vi "位置显示.vi"(5 "right":dbl=1152.0, 7 "left":dbl=846.0, 8 "error in (no error) 2":errorcluster, 10 "簇":T2, 11 "Image in":T1(plugin-control)) -> (0 "error out":errorcluster caption="错误输出", 1 "左":dbl, 2 "右":dbl, 3 "Image out":T1(plugin-control), 4 "x或y？":bool)   [LabVIEW 2017]
panel:
  out "line start X":dbl
  out "x/y":dbl
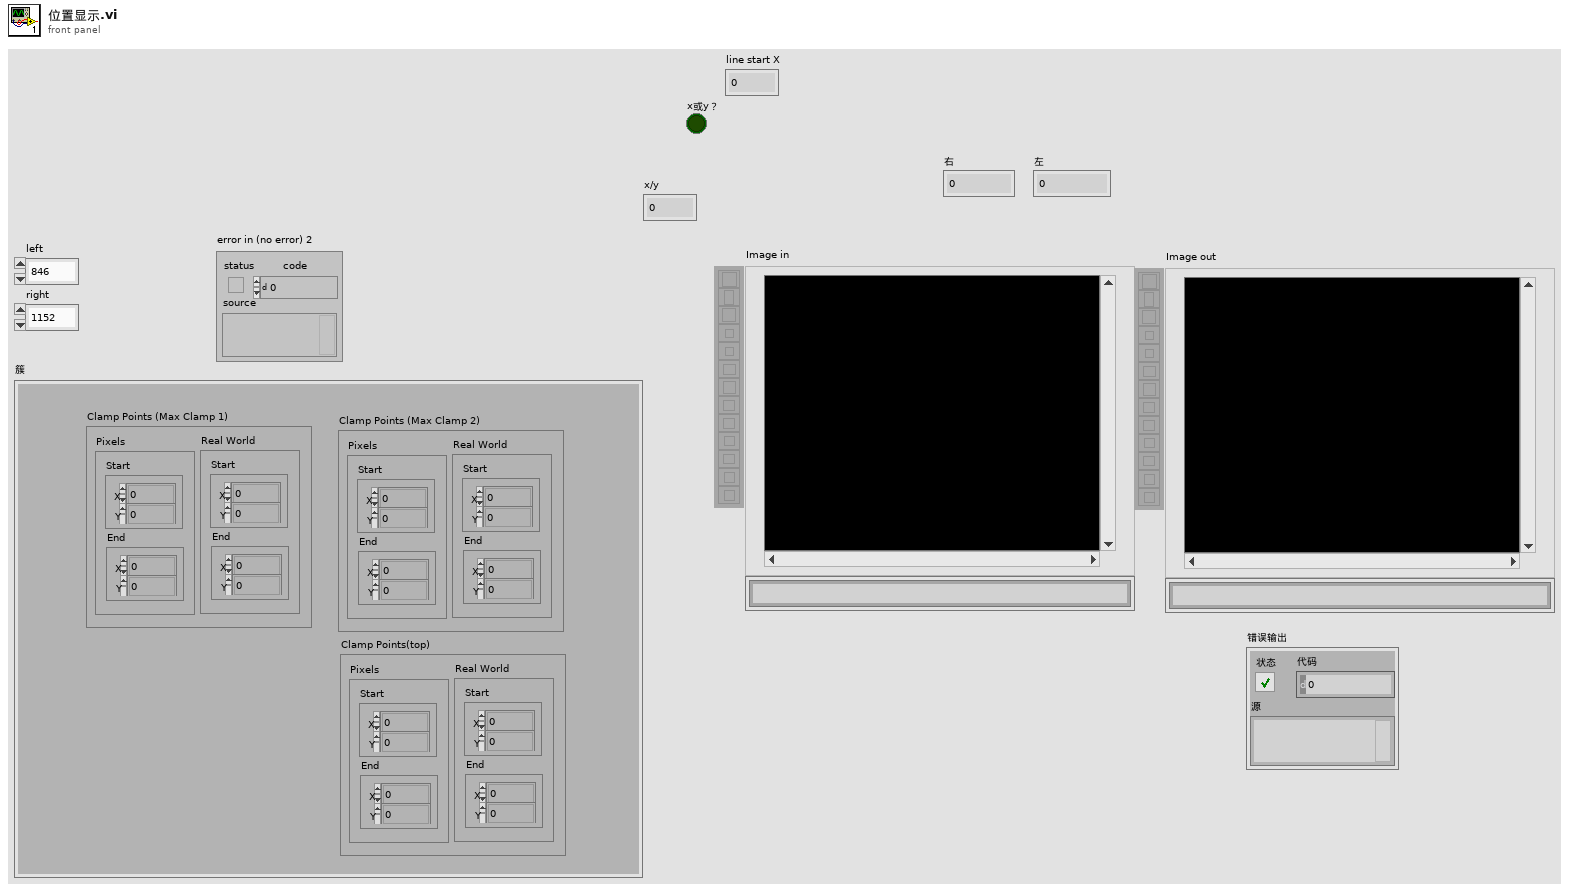
[diagram p1: front panel]
types:
  T1 = typedef "IMAQ Image.ctl" = refnum<image>
  T2 = cluster{"Clamp Points (Max Clamp 1)":cluster{"Pixels ":cluster{"Start":cluster{"X":dbl, "Y":dbl}, "End":cluster{"X":dbl, "Y":dbl}}, "Real World":cluster{"Start":cluster{"X":dbl, "Y":dbl}, "End":cluster{"X":dbl, "Y":dbl}}}, "Clamp Points (Max Clamp 2)":cluster{"Pixels ":cluster{"Start":cluster{"X":dbl, "Y":dbl}, "End":cluster{"X":dbl, "Y":dbl}}, "Real World":cluster{"Start":cluster{"X":dbl, "Y":dbl}, "End":cluster{"X":dbl, "Y":dbl}}}, "Clamp Points(top)":cluster{"Pixels ":cluster{"Start":cluster{"X":dbl, "Y":dbl}, "End":cluster{"X":dbl, "Y":dbl}}, "Real World":cluster{"Start":cluster{"X":dbl, "Y":dbl}, "End":cluster{"X":dbl, "Y":dbl}}}}
  T3 = cluster{"Pixels ":cluster{"Start":cluster{"X":dbl, "Y":dbl}, "End":cluster{"X":dbl, "Y":dbl}}, "Real World":cluster{"Start":cluster{"X":dbl, "Y":dbl}, "End":cluster{"X":dbl, "Y":dbl}}}
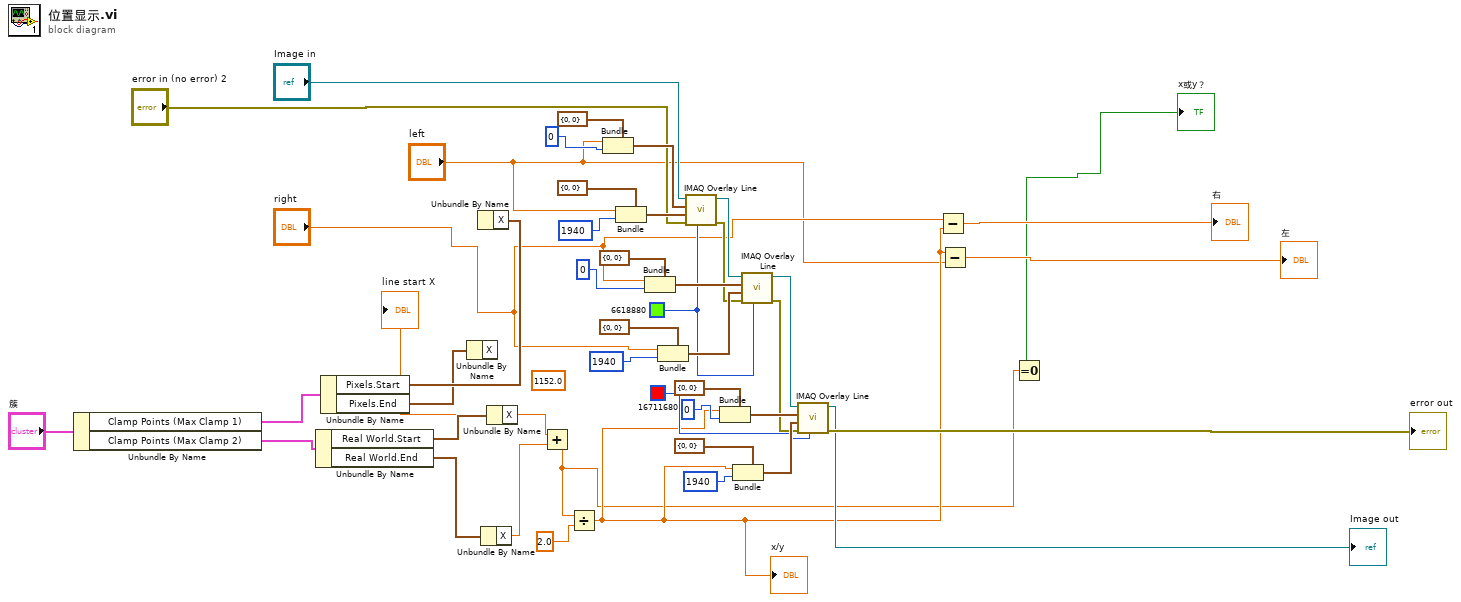
[diagram p0: block diagram]
diagram:
  (unwired) 1152.0 ("X")
  w26 = u32 6618880 ("Color")
  n1 = Unbundle By Name("簇") -> ("Clamp Points (Max Clamp 1)"=w15:T3, "Clamp Points (Max Clamp 2)"=w8:T3)
  n2 = Unbundle By Name(w8) -> ("Real World.Start"=w37:cluster{"X":dbl, "Y":dbl}, "Real World.End"=w34:cluster{"X":dbl, "Y":dbl})
  n3 = Unbundle By Name(w15) -> ("Pixels.Start"=w45:cluster{"X":dbl, "Y":dbl}, "Pixels.End"=w40:cluster{"X":dbl, "Y":dbl})
  n4 = Unbundle By Name(w40) -> ()  [unwired: 1 out]
  n5 = Unbundle By Name(w45) -> ()  [unwired: 1 out]
  n6 = Unbundle By Name(w34) -> ("X"=w24:dbl)
  n7 = Unbundle By Name(w37) -> ("X"=w25:dbl)
  "line start X" <- w25
  n8 = Add(x=w25, y=w24) -> (x+y=w2:dbl)
  n9 = Divide(x=w2, y=2.0) -> (x/y=w5:dbl)
  "x/y" <- w5
  n10 = Bundle(cluster=cluster{"X":i32, "Y":i32} {"X"=0, "Y"=0} ("End Point"), "X"="left", "Y"=0) -> (w32:cluster{"X":i32, "Y":i32})
  n11 = Bundle(cluster=cluster{"X":i32, "Y":i32} {"X"=0, "Y"=0} ("End Point"), "X"="left", "Y"=1940) -> (w42:cluster{"X":i32, "Y":i32})
  n12 = Bundle(cluster=cluster{"X":i32, "Y":i32} {"X"=0, "Y"=0} ("End Point"), "X"="right", "Y"=0) -> (w30:cluster{"X":i32, "Y":i32})
  n13 = Bundle(cluster=cluster{"X":i32, "Y":i32} {"X"=0, "Y"=0} ("End Point"), "X"="right", "Y"=1940) -> (w38:cluster{"X":i32, "Y":i32})
  n14 = call "IMAQ Overlay Line"("Color"=w26, "error in (no error)"="error in (no error) 2", "End Point"=w42, "Start Point"=w32, "Image"="Image in") -> ("error out"=w19:errorcluster, "Image Out"=w41:T1)  [unwired: 5 in]
  n15 = Bundle(cluster=cluster{"X":i32, "Y":i32} {"X"=0, "Y"=0} ("End Point"), "X"=w5, "Y"=0) -> (w28:cluster{"X":i32, "Y":i32})
  n16 = Bundle(cluster=cluster{"X":i32, "Y":i32} {"X"=0, "Y"=0} ("End Point"), "X"=w5, "Y"=1940) -> (w36:cluster{"X":i32, "Y":i32})
  n17 = call "IMAQ Overlay Line"("Color"=w26, "error in (no error)"=w19, "End Point"=w38, "Start Point"=w30, "Image"=w41) -> ("error out"=w18:errorcluster, "Image Out"=w35:T1)  [unwired: 5 in]
  n18 = call "IMAQ Overlay Line"("Color"=u32 16711680, "error in (no error)"=w18, "End Point"=w36, "Start Point"=w28, "Image"=w35) -> ("error out"=→"error out":errorcluster, "Image Out"=→"Image out":T1)  [unwired: 5 in]
  n19 = Subtract(x="right", y=w5) -> (x-y=→"右":dbl)
  n20 = Subtract(x=w5, y="left") -> (x-y=→"左":dbl)
  n21 = Equal To 0?(x=w2) -> (x = 0?=→"x或y？":bool)
